vi "Read N Records 4xI16.vi"(7 "Timeout (s)":dbl=10.0, 8 "error in":errorcluster, 11 "FPGA VI Reference In":refnum<k20>) -> (0 "error out":errorcluster, 1 "Channel 1 Records":i16[][](array[numeric]), 2 "Channel 0 Records":i16[][](array[numeric]), 3 "FPGA VI Reference Out":refnum<k20>, 4 "Elements Remaining":u32, 6 "Records Done":u32)   [LabVIEW 2012]
panel:
  out "Num I16s":u32
  out "Num U64s":u32
  out "Records to Acquire":u32
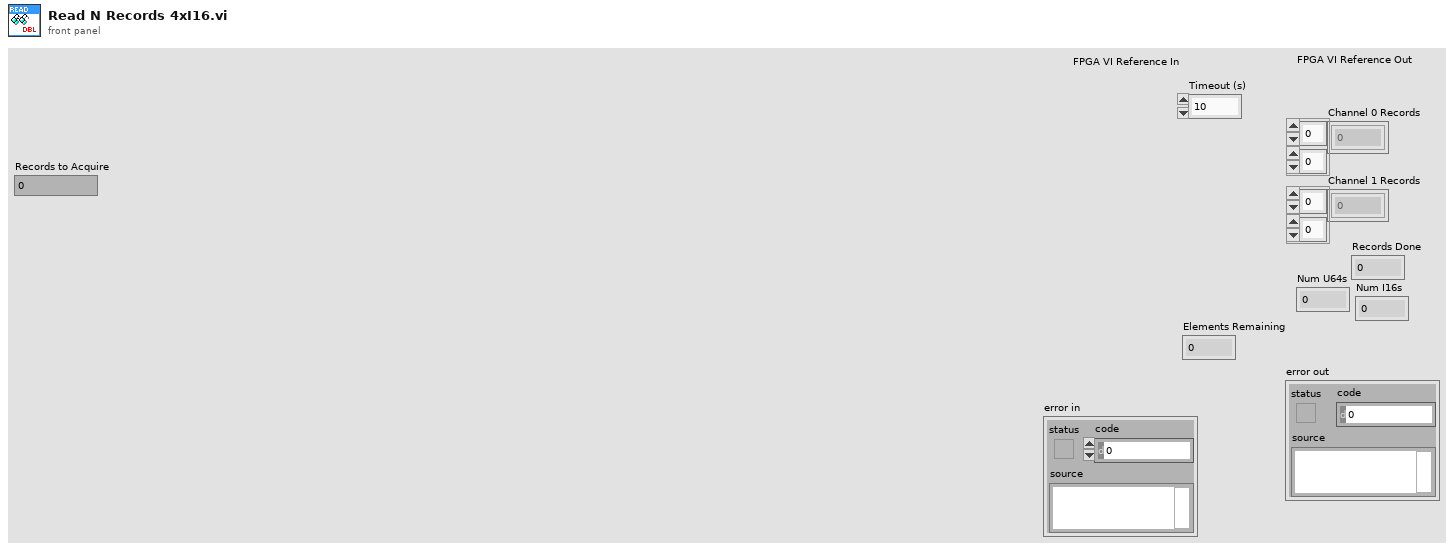
[diagram p1: front panel]
types:
  T1 = cluster{"DRAM Write Ticks":u16, "DRAM Read Ticks":u16}
  T2 = cluster{"write grant time (clocks)":u16, "read grant time (clocks)":u16}
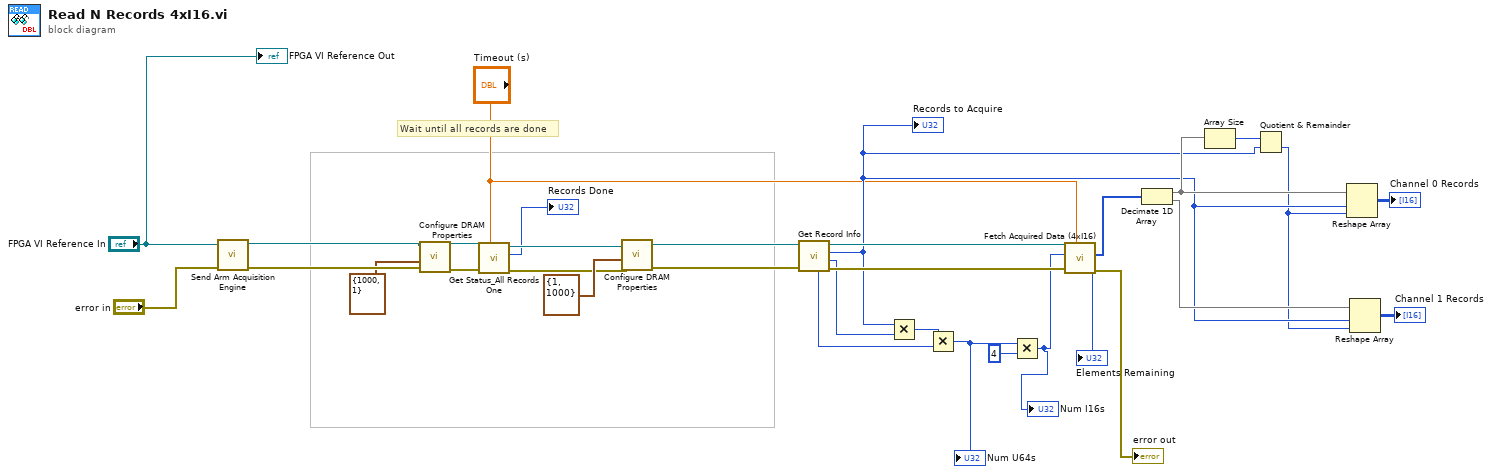
[diagram p0: block diagram]
diagram:
  # "Wait until all records are done"
  n1 = call <userlib>:"Send Arm Acquisition Engine.vi"("error in"="error in", "FPGA VI Reference In"="FPGA VI Reference In") -> ("error out"=w31:errorcluster, "FPGA VI Reference Out"=w32:refnum<k20>)  [unwired: 8 in]
  n2 = call <userlib>:"Configure DRAM Properties.vi"("error in"=w31, "DRAM Duty Cycle"=T2 {"write grant time (clocks)"=1000, "read grant time (clocks)"=1} ("DRAM Arbiter Config"), "FPGA VI Reference In"=w32) -> ("error out"=w27:errorcluster, "FPGA VI Reference Out"=w28:refnum<k20>)  [unwired: 7 in]
  n3 = call <userlib>:"Get Status_All Records One.vi"("Timeout (s)"="Timeout (s)", "error in"=w27, "FPGA VI Reference In"=w28) -> ("error out"=w26:errorcluster, "Records Done"=→"Records Done":u32, "FPGA VI Reference Out"=w25:refnum<k20>)  [unwired: 6 in]
  n4 = call <userlib>:"Configure DRAM Properties.vi"("error in"=w26, "DRAM Duty Cycle"=T1 {"DRAM Write Ticks"=1, "DRAM Read Ticks"=1000}, "FPGA VI Reference In"=w25) -> ("error out"=w23:errorcluster, "FPGA VI Reference Out"=w24:refnum<k20>)  [unwired: 7 in]
  n5 = call <userlib>:"Get Record Info.vi"("error in"=w23, "FPGA VI Reference In"=w24) -> ("error out"=w22:errorcluster, "Record Length"=w14:u32, "Records to Acquire"=w16:u32, "FPGA VI Reference Out"=w21:refnum<k20>, "Num of Channels"=w7:u32)  [unwired: 5 in]
  "Records to Acquire" <- w16
  n6 = Multiply(x=w16, y=w14) -> (x*y=w8:u32)
  n7 = Multiply(x=w8, y=w7) -> (x*y=w3:u32)
  "Num U64s" <- w3
  n8 = Multiply(x=w3, y=u32 4) -> (x*y=w1:u32)
  "Num I16s" <- w1
  n9 = call <userlib>:"Fetch Acquired Data (4xI16).vi"("Timeout (s)"="Timeout (s)", "error out"=w22, "Samples"=w1, "FPGA Ref In"=w21) -> ("error out"=→"error out":errorcluster, "Data"=w19:i16[], "Elements Remaining"=→"Elements Remaining":u32)  [unwired: 4 in, 1 out]
  n10 = Decimate 1D Array(w19) -> (w18:i16[], w20:i16[])
  n11 = Array Size(array=w18) -> (size(s)=w17:i32)
  n12 = Quotient & Remainder(x=w17, y=w16) -> (floor(x/y)=w15:u32)  [unwired: 1 out]
  n13 = Reshape Array(w18, w16, w15) -> (→"Channel 0 Records":i16[][])
  n14 = Reshape Array(w20, w16, w15) -> (→"Channel 1 Records":i16[][])
  "FPGA VI Reference Out" <- "FPGA VI Reference In"
